vi "Handle Command.vi"(8 "error in (no error)":errorcluster, 9 "Data":variant, 10 "Command":string, 11 "Instrument.VRM in":refnum<class "Instrument.OxfordVRM.lvclass">) -> (0 "error out":errorcluster, 1 "Processed Data":variant, 2 "Command":string, 3 "Instrument.VRM out":refnum<class "Instrument.OxfordVRM.lvclass">)   [LabVIEW 2019, in "Instrument.OxfordVRM.lvclass"]
uses:
  Instrument.OxfordVRM.lvclass
  Typedefs/Instrument.VRM.Commands-enum.ctl
  Typedefs/VRM Action-Axis--Cluster.ctl
  <instrlib>/Mercury iXX/Public/Libraries/Magnet/Controls/PSU Actions.ctl
  Typedefs/VRM Magnet Axis--Enum.ctl
  <userlib>/LevyLab/Levylab Instruments/Instrument Types/Cryostat/Typedefs/Magnet Axis--Enum.ctl
  Typedefs/VRM Targets--Cluster.ctl
  Instrument.OxfordVRM.lvclass/Instrument.OxfordVRM.ctl
  Typedefs/Instrument.VRM.setMagnet-cluster.ctl
  <userlib>/LevyLab/Levylab Instruments/Instrument Types/Cryostat/Instrument.Cryostat.lvclass
  <instrlib>/Mercury iXX/Public/Libraries/Magnet.lvlib
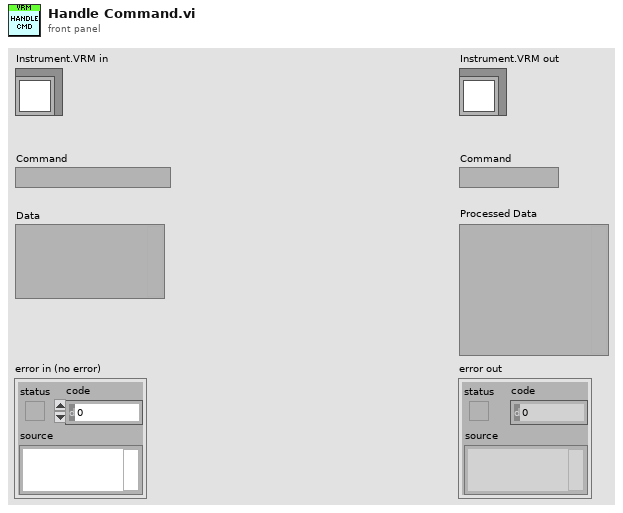
[diagram p1: front panel]
types:
  T1 = typedef "Instrument.OxfordVRM.lvclass/Instrument.VRM.Commands-enum.ctl" = enum16{"setAction", "setTarget", "setMagnetField", "getStatus", "getTarget", "getMagnetField"}
  T2 = typedef "Instrument.OxfordVRM.lvclass/VRM Action-Axis--Cluster.ctl" = cluster{"PSU Act Stat":T3, "Axis":T4}
  T3 = typedef "Mercury iXX.lvlib/Magnet.lvlib/PSU Actions.ctl" = string
  T4 = typedef "Instrument.OxfordVRM.lvclass/VRM Magnet Axis--Enum.ctl" = enum16{"Z", "X", "Y", "ALL"}
  T5 = typedef "Instrument.Cryostat.lvclass/Magnet Axis--Enum.ctl" = enum16{"Z", "X", "Y"}
  T6 = typedef "Instrument.OxfordVRM.lvclass/VRM Targets--Cluster.ctl" = cluster{"Field (T)":dbl[], "Field Rate (T/min)":dbl, "Axis":T4}
  T7 = typedef "Instrument.OxfordVRM.lvclass/Instrument.VRM.setMagnet-cluster.ctl" = cluster{"Target":T6}
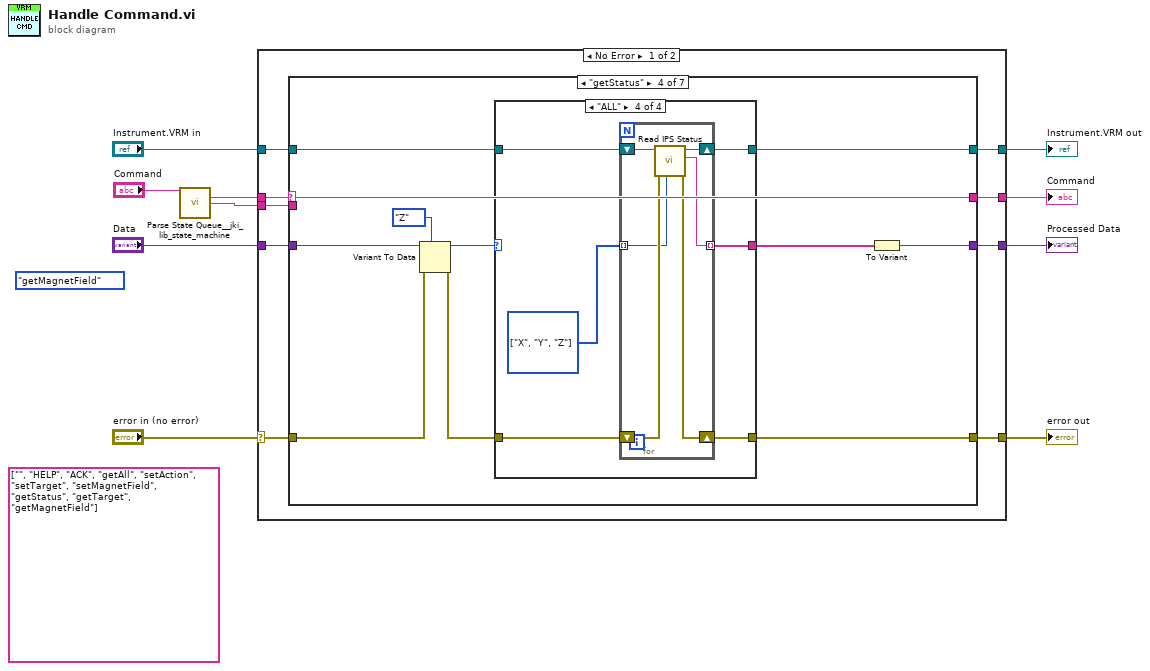
[diagram p0: block diagram]
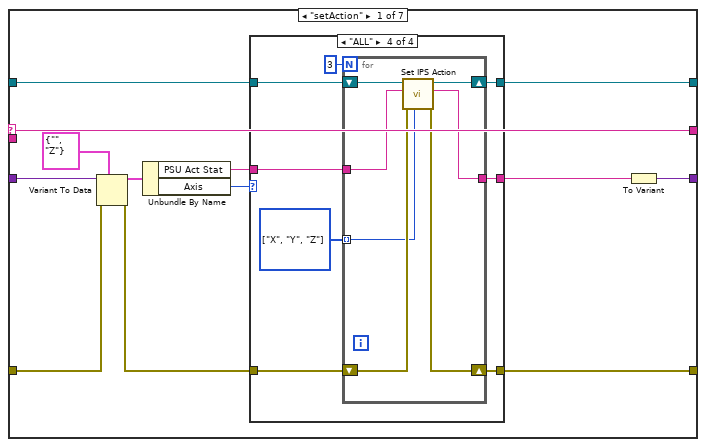
[diagram p2: hidden frame]
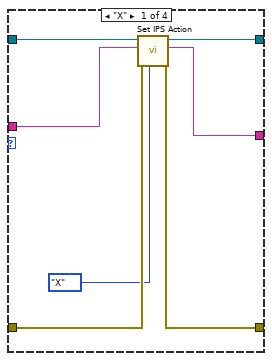
[diagram p3: hidden frame]
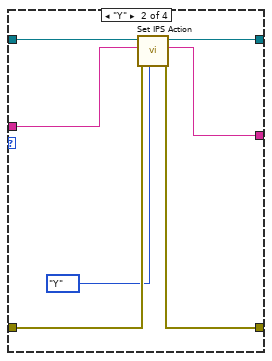
[diagram p4: hidden frame]
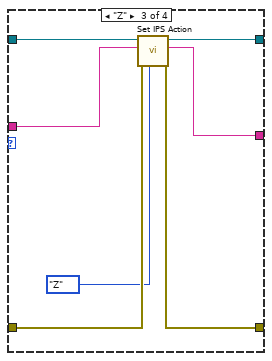
[diagram p5: hidden frame]
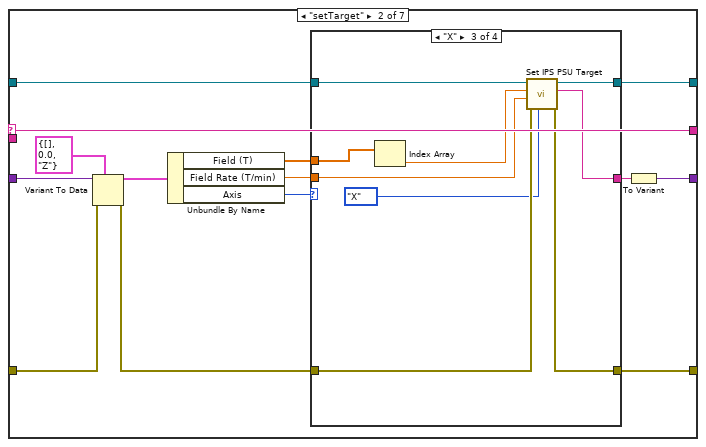
[diagram p6: hidden frame]
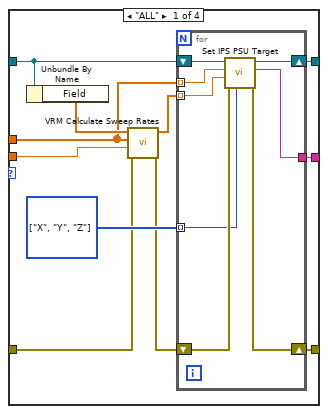
[diagram p7: hidden frame]
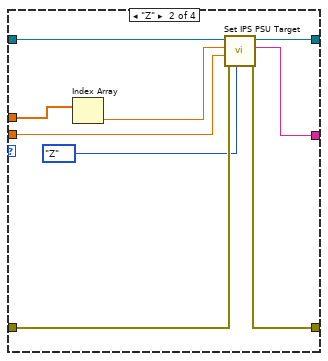
[diagram p8: hidden frame]
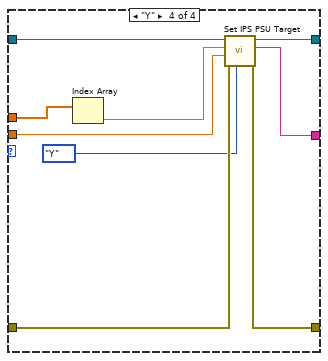
[diagram p9: hidden frame]
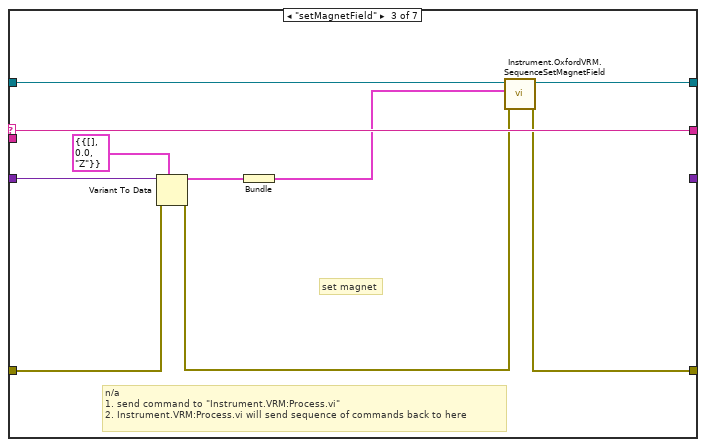
[diagram p10: hidden frame]
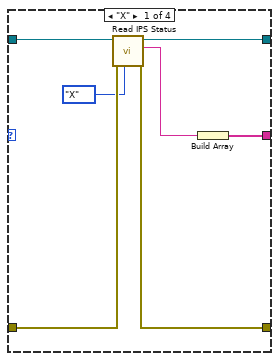
[diagram p11: hidden frame]
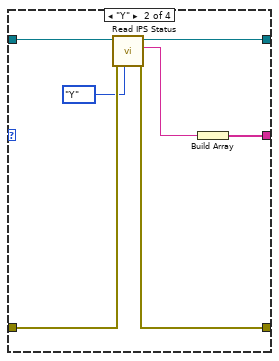
[diagram p12: hidden frame]
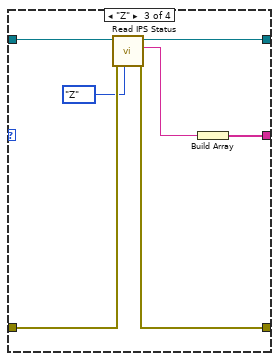
[diagram p13: hidden frame]
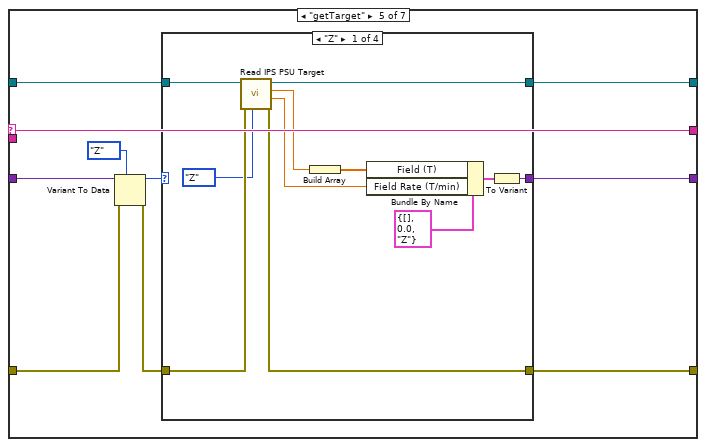
[diagram p14: hidden frame]
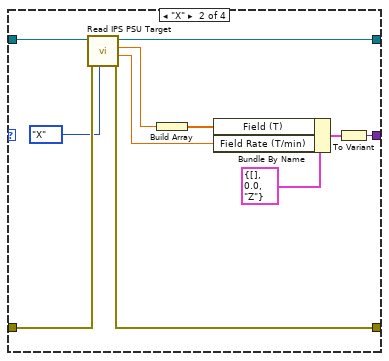
[diagram p15: hidden frame]
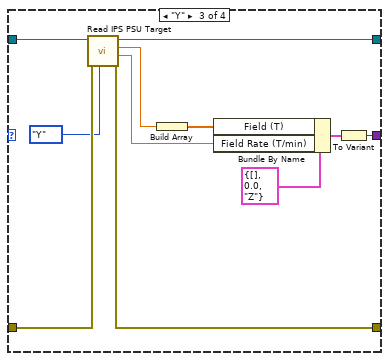
[diagram p16: hidden frame]
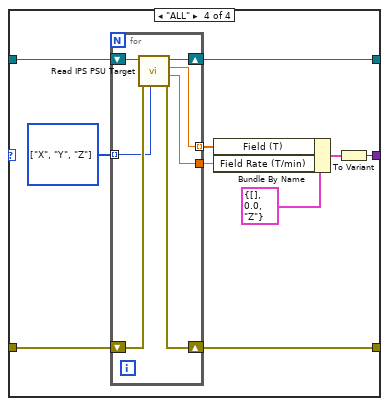
[diagram p17: hidden frame]
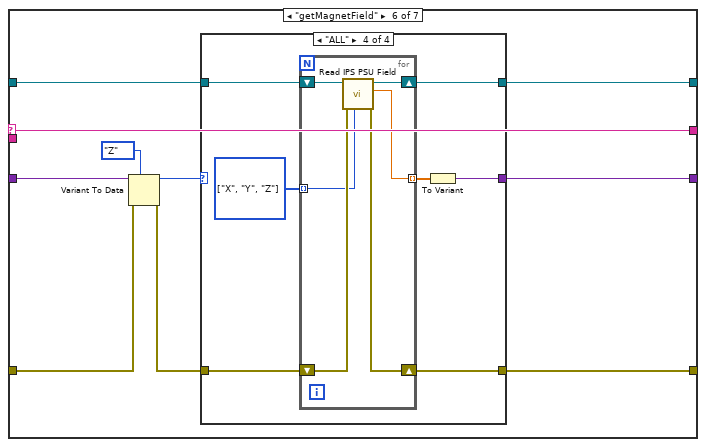
[diagram p18: hidden frame]
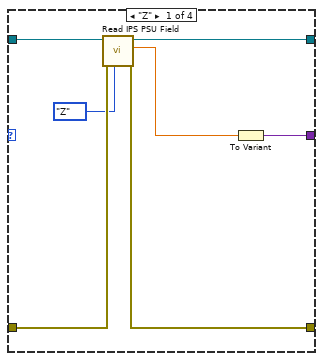
[diagram p19: hidden frame]
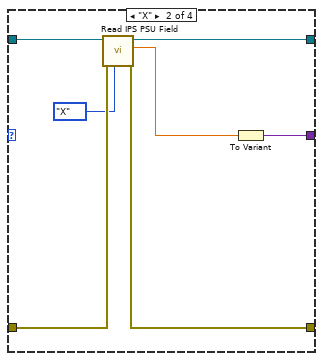
[diagram p20: hidden frame]
diagram:
  (unwired) Instrument.VRM.Commands-enum."getMagnetField" ("Commands")
  (unwired) string[] ["", "HELP", "ACK", "getAll", "setAction", "setTarget", "setMagnetField", "getStatus", "getTarget", "getMagnetField"] ("Commands")
  n1 = call <vilib>:"Parse State Queue__jki_lib_state_machine.vi"("State Queue"="Command") -> ("Current State"=w2:string, "Arguments"=w1:string)  [unwired: 12 in, 1 out]
  n2 = case shown="No Error" "error in (no error)" {
    selector: "error in (no error)" -> [w14 w295]
    tunnel: [w13 w295] -> w10
    tunnel: [w19 _] -> w9
    tunnel: [w18 _] -> w8
    tunnel: [w17 w296] -> w7
    tunnel: "Data" -> [w16 _]
    tunnel: w2 -> [w11 _]
    tunnel: "Instrument.VRM in" -> [w15 w296]
    tunnel: w1 -> [w12 _]
    frame No Error {
      n3 = case shown="\"getStatus\"" w11 {
        selector: w11 -> [w32 w82 w138 w149 w192 w252 w287]
        tunnel: [w27 w78 _ w148 w191 w251 w289] -> w19
        tunnel: [w32 w82 w138 w149 w192 w252 w294] -> w18
        tunnel: [w30 w80 w133 w145 w189 w249 w293] -> w17
        tunnel: w16 -> [w26 w77 w137 w143 w186 w246 w288]
        tunnel: w15 -> [w31 w81 w134 w146 w188 w250 w292]
        tunnel: w14 -> [w23 w74 w136 w142 w185 w245 w291]
        tunnel: [w29 w79 w129 w140 w190 w248 w290] -> w13
        tunnel: w12 -> [_ _ _ _ _ _ _]
        frame "setAction" {
          n4 = Variant To Data(error in=w23, type=T2 {"PSU Act Stat"="", "Axis"=enum."Z"} ("Action"), Variant=w26) -> (data=w24:T2, error out=w22:errorcluster)
          n5 = Unbundle By Name(w24) -> ("PSU Act Stat"=w21:T3, "Axis"=w20:T4)
          n6 = case shown="\"ALL\"" w20 {
            tunnel: w31 -> [w39 w46 w53 w61]
            tunnel: [w38 w45 w52 w60] -> w30
            tunnel: [w37 w44 w51 w59] -> w29
            tunnel: [w36 w43 w50 w58] -> w28
            tunnel: w22 -> [w35 w42 w49 w57]
            tunnel: w21 -> [w34 w41 w48 w56]
            frame "X" {
              n7 = call "Set IPS Action.vi"("Axis"=Magnet_Axis--Enum."X", "error in (no error)"=w35, "PSU Act Stat"=w34, "Instrument.OxfordVRM in"=w39) -> ("error out"=w37:errorcluster, "Response"=w36:string, "Instrument.OxfordVRM out"=w38:refnum<class "Instrument.OxfordVRM.lvclass">)  [unwired: 5 in]
            }
            frame "Y" {
              n8 = call "Set IPS Action.vi"("Axis"=Magnet_Axis--Enum."Y", "error in (no error)"=w42, "PSU Act Stat"=w41, "Instrument.OxfordVRM in"=w46) -> ("error out"=w44:errorcluster, "Response"=w43:string, "Instrument.OxfordVRM out"=w45:refnum<class "Instrument.OxfordVRM.lvclass">)  [unwired: 5 in]
            }
            frame "Z" {
              n9 = call "Set IPS Action.vi"("Axis"=Magnet_Axis--Enum."Z", "error in (no error)"=w49, "PSU Act Stat"=w48, "Instrument.OxfordVRM in"=w53) -> ("error out"=w51:errorcluster, "Response"=w50:string, "Instrument.OxfordVRM out"=w52:refnum<class "Instrument.OxfordVRM.lvclass">)  [unwired: 5 in]
            }
            frame "ALL" {
              w54 = T5[] [enum."X", enum."Y", enum."Z"] items=["Z", "X", "Y"]
              n10 = for {
                N: 3 -> [_]
                tunnel: [w65] -> w58
                tunnel: w56 -> [w63]
                shift-right: [w67] -> w60
                shift-left: w61 -> [w68]
                shift-right: [w66] -> w59
                shift-left: w57 -> [w64]
                tunnel: w54 -> [w62] mode=indexing
                n11 = call "Set IPS Action.vi"("Axis"=w62, "error in (no error)"=w64, "PSU Act Stat"=w63, "Instrument.OxfordVRM in"=w68) -> ("error out"=w66:errorcluster, "Response"=w65:string, "Instrument.OxfordVRM out"=w67:refnum<class "Instrument.OxfordVRM.lvclass">)  [unwired: 5 in]
              }
            }
          }
          n12 = To Variant(anything=w28) -> (Variant=w27:variant)
        }
        frame "setTarget" {
          n13 = Variant To Data(error in=w74, type=T6 {"Field (T)"=[], "Field Rate (T/min)"=0.0, "Axis"=enum."Z"} ("Targets"), Variant=w77) -> (data=w75:T6, error out=w73:errorcluster)
          n14 = Unbundle By Name(w75) -> ("Field (T)"=w70:dbl[], "Field Rate (T/min)"=w71:dbl, "Axis"=w69:T4)
          n15 = case shown="\"X\"" w69 {
            tunnel: w81 -> [w89 w110 w119 w128]
            tunnel: [w93 w109 w118 w127] -> w80
            tunnel: [w92 w108 w117 w126] -> w79
            tunnel: w73 -> [w85 w107 w116 w125]
            tunnel: [w91 w106 w115 w124] -> w72
            tunnel: w71 -> [w83 w105 w114 w123]
            tunnel: w70 -> [w87 w104 w113 w122]
            frame "ALL" {
              w90 = T5[] [enum."X", enum."Y", enum."Z"] items=["Z", "X", "Y"]
              n16 = Unbundle By Name(w89) -> ("Field"=w88:dbl[])
              n17 = call "VRM Calculate Sweep Rates.vi"("error in (no error)"=w85, "Sweep rate (T/min)"=w83, "Target Field (T)"=w87, "Initial Field (T)"=w88) -> ("error out"=w84:errorcluster, "Sweep Rate Field (T/min)"=w86:dbl[])  [unwired: 5 in, 1 out]
              n18 = for {
                tunnel: [w97] -> w91
                tunnel: w86 -> [w96] mode=indexing
                shift-right: [w100] -> w93
                shift-left: w89 -> [w101]
                shift-right: [w99] -> w92
                shift-left: w84 -> [w98]
                tunnel: w87 -> [w95] mode=indexing
                tunnel: w90 -> [w94] mode=indexing
                n19 = call "Set IPS PSU Target.vi"("Axis"=w94, "error in (no error)"=w98, "Target Field Rate (T/min)"=w96, "Target Field (T)"=w95, "Instrument.OxfordVRM in"=w101) -> ("error out"=w99:errorcluster, "Response"=w97:string, "Instrument.OxfordVRM out"=w100:refnum<class "Instrument.OxfordVRM.lvclass">)  [unwired: 4 in]
              }
            }
            frame "Z" {
              n20 = Index Array(array=w104) -> (element=w103:dbl)  [unwired: 1 in]
              n21 = call "Set IPS PSU Target.vi"("Axis"=Magnet_Axis--Enum."Z", "error in (no error)"=w107, "Target Field Rate (T/min)"=w105, "Target Field (T)"=w103, "Instrument.OxfordVRM in"=w110) -> ("error out"=w108:errorcluster, "Response"=w106:string, "Instrument.OxfordVRM out"=w109:refnum<class "Instrument.OxfordVRM.lvclass">)  [unwired: 4 in]
            }
            frame "X" {
              n22 = Index Array(array=w113) -> (element=w112:dbl)  [unwired: 1 in]
              n23 = call "Set IPS PSU Target.vi"("Axis"=Magnet_Axis--Enum."X", "error in (no error)"=w116, "Target Field Rate (T/min)"=w114, "Target Field (T)"=w112, "Instrument.OxfordVRM in"=w119) -> ("error out"=w117:errorcluster, "Response"=w115:string, "Instrument.OxfordVRM out"=w118:refnum<class "Instrument.OxfordVRM.lvclass">)  [unwired: 4 in]
            }
            frame "Y" {
              n24 = Index Array(array=w122) -> (element=w121:dbl)  [unwired: 1 in]
              n25 = call "Set IPS PSU Target.vi"("Axis"=Magnet_Axis--Enum."Y", "error in (no error)"=w125, "Target Field Rate (T/min)"=w123, "Target Field (T)"=w121, "Instrument.OxfordVRM in"=w128) -> ("error out"=w126:errorcluster, "Response"=w124:string, "Instrument.OxfordVRM out"=w127:refnum<class "Instrument.OxfordVRM.lvclass">)  [unwired: 4 in]
            }
          }
          n26 = To Variant(anything=w72) -> (Variant=w78:variant)
        }
        frame "setMagnetField" {
          # "set magnet"
          # "n/a\n1. send command to \"Instrument.VRM:Process.vi\"\n2. Instrument.VRM:Process.vi will send sequence of commands back to here"
          n27 = Variant To Data(error in=w136, type=T7 {"Target"={"Field (T)"=[], "Field Rate (T/min)"=0.0, "Axis"=enum."Z"}} ("output cluster"), Variant=w137) -> (data=w131:T7, error out=w130:errorcluster)
          n28 = Bundle("output cluster"=w131) -> (w132:cluster{"output cluster":T7})  [unwired: 1 in]
          n29 = call "Instrument.OxfordVRM.SequenceSetMagnetField.vi"("error in (no error)"=w130, "Set Magnet Field"=w132, "Instrument.Oxford1820"=w134) -> ("error out"=w129:errorcluster, "Instrument.Oxford1820 out"=w133:refnum<class "Instrument.OxfordVRM.lvclass">)  [unwired: 7 in]
        }
        frame "getStatus" {
          n30 = Variant To Data(error in=w142, type=VRM_Magnet_Axis--Enum."Z" ("Target.Axis"), Variant=w143) -> (data=w139:T4, error out=w141:errorcluster)
          n31 = case shown="\"ALL\"" w139 {
            tunnel: [w151 w158 w165 w172] -> w147
            tunnel: w146 -> [w155 w162 w169 w176]
            tunnel: [w154 w161 w168 w175] -> w145
            tunnel: w141 -> [w153 w160 w167 w174]
            tunnel: [w152 w159 w166 w173] -> w140
            frame "X" {
              n32 = call "Read IPS Status.vi"("Axis"=Magnet_Axis--Enum."X", "error in (no error)"=w153, "Instrument.OxfordVRM in"=w155) -> ("error out"=w152:errorcluster, "Status"=w156:string, "Instrument.OxfordVRM out"=w154:refnum<class "Instrument.OxfordVRM.lvclass">)  [unwired: 6 in]
              n33 = Build Array(w156) -> (w151:string[])
            }
            frame "Y" {
              n34 = call "Read IPS Status.vi"("Axis"=Magnet_Axis--Enum."Y", "error in (no error)"=w160, "Instrument.OxfordVRM in"=w162) -> ("error out"=w159:errorcluster, "Status"=w163:string, "Instrument.OxfordVRM out"=w161:refnum<class "Instrument.OxfordVRM.lvclass">)  [unwired: 6 in]
              n35 = Build Array(w163) -> (w158:string[])
            }
            frame "Z" {
              n36 = call "Read IPS Status.vi"("Axis"=Magnet_Axis--Enum."Z", "error in (no error)"=w167, "Instrument.OxfordVRM in"=w169) -> ("error out"=w166:errorcluster, "Status"=w170:string, "Instrument.OxfordVRM out"=w168:refnum<class "Instrument.OxfordVRM.lvclass">)  [unwired: 6 in]
              n37 = Build Array(w170) -> (w165:string[])
            }
            frame "ALL" {
              w171 = T5[] [enum."X", enum."Y", enum."Z"] items=["Z", "X", "Y"]
              n38 = for {
                tunnel: [w178] -> w172 mode=indexing
                shift-right: [w181] -> w175
                shift-left: w176 -> [w182]
                shift-right: [w179] -> w173
                shift-left: w174 -> [w180]
                tunnel: w171 -> [w177] mode=indexing
                n39 = call "Read IPS Status.vi"("Axis"=w177, "error in (no error)"=w180, "Instrument.OxfordVRM in"=w182) -> ("error out"=w179:errorcluster, "Status"=w178:string, "Instrument.OxfordVRM out"=w181:refnum<class "Instrument.OxfordVRM.lvclass">)  [unwired: 6 in]
              }
            }
          }
          n40 = To Variant(anything=w147) -> (Variant=w148:variant)
        }
        frame "getTarget" {
          n41 = Variant To Data(error in=w185, type=VRM_Magnet_Axis--Enum."Z" ("Target.Axis"), Variant=w186) -> (data=w183:T4, error out=w184:errorcluster)
          n42 = case shown="\"Z\"" w183 {
            tunnel: [w203 w214 w225 w235] -> w191
            tunnel: [w200 w211 w222 w232] -> w190
            tunnel: [w199 w210 w221 w231] -> w189
            tunnel: w188 -> [w198 w209 w220 w230]
            tunnel: w184 -> [w197 w208 w219 w229]
            frame "Z" {
              n43 = call "Read IPS PSU Target.vi"("Axis"=Magnet_Axis--Enum."Z", "error in (no error)"=w197, "Instrument.OxfordVRM in"=w198) -> ("error out"=w200:errorcluster, "Target Field Rate (T/min)"=w195:dbl, "Target Field (T)"=w194:dbl, "Instrument.OxfordVRM out"=w199:refnum<class "Instrument.OxfordVRM.lvclass">)  [unwired: 5 in]
              n44 = Build Array(w194) -> (w193:dbl[])
              n45 = Bundle By Name(cluster=T6 {"Field (T)"=[], "Field Rate (T/min)"=0.0, "Axis"=enum."Z"} ("Target"), "Field (T)"=w193, "Field Rate (T/min)"=w195) -> (w202:T6)
              n46 = To Variant(anything=w202) -> (Variant=w203:variant)
            }
            frame "X" {
              n47 = call "Read IPS PSU Target.vi"("Axis"=Magnet_Axis--Enum."X", "error in (no error)"=w208, "Instrument.OxfordVRM in"=w209) -> ("error out"=w211:errorcluster, "Target Field Rate (T/min)"=w206:dbl, "Target Field (T)"=w205:dbl, "Instrument.OxfordVRM out"=w210:refnum<class "Instrument.OxfordVRM.lvclass">)  [unwired: 5 in]
              n48 = Build Array(w205) -> (w204:dbl[])
              n49 = Bundle By Name(cluster=T6 {"Field (T)"=[], "Field Rate (T/min)"=0.0, "Axis"=enum."Z"} ("Target"), "Field (T)"=w204, "Field Rate (T/min)"=w206) -> (w213:T6)
              n50 = To Variant(anything=w213) -> (Variant=w214:variant)
            }
            frame "Y" {
              n51 = call "Read IPS PSU Target.vi"("Axis"=Magnet_Axis--Enum."Y", "error in (no error)"=w219, "Instrument.OxfordVRM in"=w220) -> ("error out"=w222:errorcluster, "Target Field Rate (T/min)"=w217:dbl, "Target Field (T)"=w216:dbl, "Instrument.OxfordVRM out"=w221:refnum<class "Instrument.OxfordVRM.lvclass">)  [unwired: 5 in]
              n52 = Build Array(w216) -> (w215:dbl[])
              n53 = Bundle By Name(cluster=T6 {"Field (T)"=[], "Field Rate (T/min)"=0.0, "Axis"=enum."Z"} ("Target"), "Field (T)"=w215, "Field Rate (T/min)"=w217) -> (w224:T6)
              n54 = To Variant(anything=w224) -> (Variant=w225:variant)
            }
            frame "ALL" {
              w226 = T5[] [enum."X", enum."Y", enum."Z"] items=["Z", "X", "Y"]
              n55 = for {
                tunnel: [w238] -> w228
                shift-right: [w241] -> w231
                shift-left: w230 -> [w240]
                shift-right: [w242] -> w232
                shift-left: w229 -> [w239]
                tunnel: [w237] -> w227 mode=indexing
                tunnel: w226 -> [w236] mode=indexing
                n56 = call "Read IPS PSU Target.vi"("Axis"=w236, "error in (no error)"=w239, "Instrument.OxfordVRM in"=w240) -> ("error out"=w242:errorcluster, "Target Field Rate (T/min)"=w238:dbl, "Target Field (T)"=w237:dbl, "Instrument.OxfordVRM out"=w241:refnum<class "Instrument.OxfordVRM.lvclass">)  [unwired: 5 in]
              }
              n57 = Bundle By Name(cluster=T6 {"Field (T)"=[], "Field Rate (T/min)"=0.0, "Axis"=enum."Z"} ("Target"), "Field (T)"=w227, "Field Rate (T/min)"=w228) -> (w234:T6)
              n58 = To Variant(anything=w234) -> (Variant=w235:variant)
            }
          }
        }
        frame "getMagnetField" {
          n59 = Variant To Data(error in=w245, type=VRM_Magnet_Axis--Enum."Z" ("Target.Axis"), Variant=w246) -> (data=w243:T4, error out=w244:errorcluster)
          n60 = case shown="\"ALL\"" w243 {
            tunnel: [w259 w266 w273 w280] -> w251
            tunnel: w250 -> [w258 w265 w272 w279]
            tunnel: [w257 w264 w271 w278] -> w249
            tunnel: [w255 w262 w269 w276] -> w248
            tunnel: w244 -> [w254 w261 w268 w275]
            frame "Z" {
              n61 = call "Read IPS PSU Field.vi"("Axis"=Magnet_Axis--Enum."Z", "error in (no error)"=w254, "Instrument.OxfordVRM in"=w258) -> ("error out"=w255:errorcluster, "Power Supply Field (T)"=w256:dbl, "Instrument.OxfordVRM out"=w257:refnum<class "Instrument.OxfordVRM.lvclass">)  [unwired: 6 in]
              n62 = To Variant(anything=w256) -> (Variant=w259:variant)
            }
            frame "X" {
              n63 = call "Read IPS PSU Field.vi"("Axis"=Magnet_Axis--Enum."X", "error in (no error)"=w261, "Instrument.OxfordVRM in"=w265) -> ("error out"=w262:errorcluster, "Power Supply Field (T)"=w263:dbl, "Instrument.OxfordVRM out"=w264:refnum<class "Instrument.OxfordVRM.lvclass">)  [unwired: 6 in]
              n64 = To Variant(anything=w263) -> (Variant=w266:variant)
            }
            frame "Y" {
              n65 = call "Read IPS PSU Field.vi"("Axis"=Magnet_Axis--Enum."Y", "error in (no error)"=w268, "Instrument.OxfordVRM in"=w272) -> ("error out"=w269:errorcluster, "Power Supply Field (T)"=w270:dbl, "Instrument.OxfordVRM out"=w271:refnum<class "Instrument.OxfordVRM.lvclass">)  [unwired: 6 in]
              n66 = To Variant(anything=w270) -> (Variant=w273:variant)
            }
            frame "ALL" {
              w274 = T5[] [enum."X", enum."Y", enum."Z"] items=["Z", "X", "Y"]
              n67 = for {
                tunnel: [w284] -> w277 mode=indexing
                shift-right: [w285] -> w278
                shift-left: w279 -> [w286]
                shift-right: [w283] -> w276
                shift-left: w275 -> [w282]
                tunnel: w274 -> [w281] mode=indexing
                n68 = call "Read IPS PSU Field.vi"("Axis"=w281, "error in (no error)"=w282, "Instrument.OxfordVRM in"=w286) -> ("error out"=w283:errorcluster, "Power Supply Field (T)"=w284:dbl, "Instrument.OxfordVRM out"=w285:refnum<class "Instrument.OxfordVRM.lvclass">)  [unwired: 6 in]
              }
              n69 = To Variant(anything=w277) -> (Variant=w280:variant)
            }
          }
        }
        frame Default {
          # "HELP, ACK, getAll"
          # "commands handled by parent go here (HELP, etc_"
          n70 = call-parent "Handle Command.vi"("error in (no error)"=w291, "Data"=w288, "Command"=w287, "Instrument in"=w292) -> ("error out"=w290:errorcluster, "Processed Data"=w289:variant, "Command"=w294:string, "Instrument out"=w293:refnum<class "Instrument.OxfordVRM.lvclass">)  [unwired: 4 in]
        }
      }
    }
    frame Error {
    }
  }
  "error out" <- w10
  "Instrument.VRM out" <- w7
  "Processed Data" <- w9
  "Command" <- w8
